vi "Get DVR for Path.vi"(8 "Error in":errorcluster, 11 "Class path":path) -> (0 "Error out":errorcluster, 3 "DVR Out":refnum<data-value>)   [LabVIEW 2020, in "Test.lvclass"]
doc: "Get class from the path and generate DVR for the class object"
uses:
  Test.lvclass
panel:
  out "Test out":refnum<class "Test.lvclass">
  in  "Test in":refnum<class "Test.lvclass">
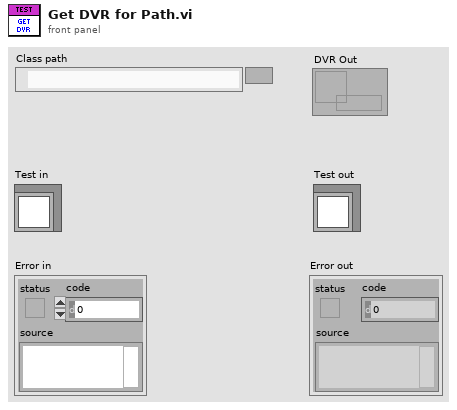
[diagram p1: front panel]
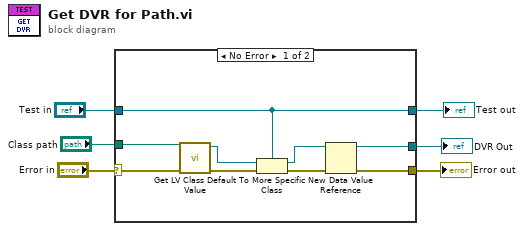
[diagram p0: block diagram]
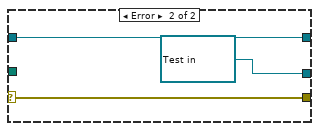
[diagram p2: hidden frame]
diagram:
  n1 = case shown="No Error" "Error in" {
    selector: "Error in" -> [w14 w18]
    tunnel: [w13 w18] -> w5
    tunnel: [w11 w17] -> w3
    tunnel: "Test in" -> [w11 w17]
    tunnel: "Class path" -> [w15 _]
    tunnel: [w7 refnum<data-value> refnum ("data value reference")] -> w1
    frame No Error {
      n2 = call <vilib>:"Get LV Class Default Value.vi"("error in (no error)"=w14, "class path"=w15) -> ("error out"=w12:errorcluster, "object"=w10:refnum<class>)  [unwired: 8 in]
      n3 = To More Specific Class(target class=w11, reference=w10, error in=w12) -> (specific class reference=w8:refnum<class "Test.lvclass">, error out=w9:errorcluster)
      n4 = New Data Value Reference(data value=w8, error in=w9) -> (data value reference=w7:refnum<data-value>, error out=w13:errorcluster)
    }
    frame Error {
    }
  }
  "Error out" <- w5
  "Test out" <- w3
  "DVR Out" <- w1
